vi "ExFileReadNDoMath.vi"() -> ()   [LabVIEW 2010]
panel:
  in  "Full File Name":path
  in  "?":bool
  in  "FileType":u32=67174400
  out "error out":errorcluster
  in  "error in (no error)":errorcluster
  # "ExReadFileNDisplay.vi\nThis example will read in a file of the\nselected data type and display all frames.\nWhen finished viewing data, make sure to\nuse the STOP button to close the display."
  # "File Types:\nSPE = 67371008\nTIF   = 67174400\nPMI  = 67436544"
  # "Browse match pattern is set to *.tif.  Modify this if different file type is needed."
  # "This will properly close\nthe image and\ndeallocate memory."
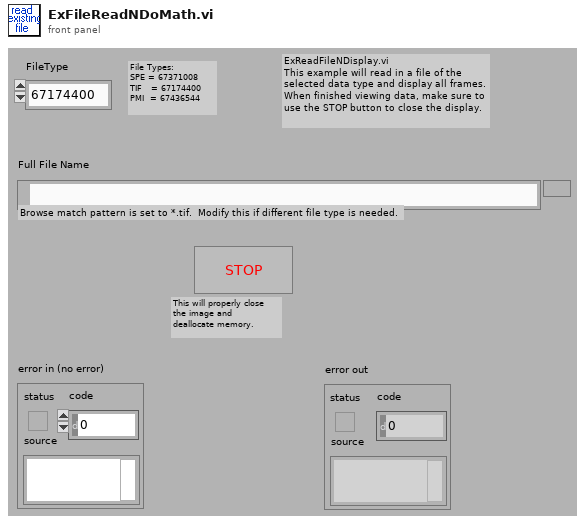
[diagram p1: front panel]
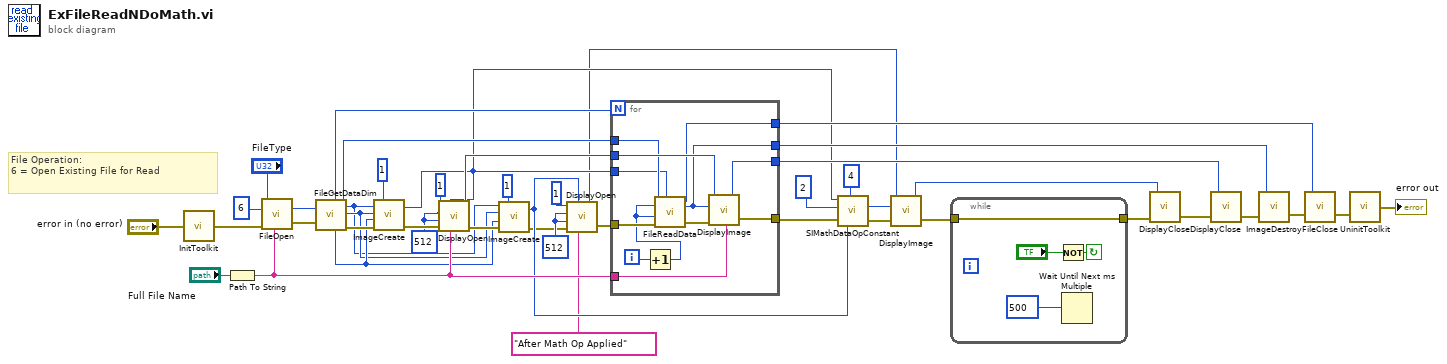
[diagram p0: block diagram]
diagram:
  w13 = 512
  w35 = 512
  # "File Operation:\n6 = Open Existing File for Read"
  n1 = call <userlib>:"InitToolkit.vi"("error in"="error in (no error)") -> ("error out"=w43:errorcluster)
  n2 = Path To String(path="Full File Name") -> (string=w23:string)
  n3 = call <userlib>:"FileOpen.vi"("error in"=w43, "File Operations"=u32 6 ("File Operation"), "FileName"=w23, "File Type"="FileType") -> ("error out"=w41:errorcluster, "File Handle"=w40:u32)
  n4 = call <userlib>:"FileGetDataDim.vi"("File Handle"=w40, "error in"=w41) -> ("Number of Frames"=w37:u32, "Data Type"=w20:u32, "File Handle"=w32:u32, "X dim"=w18:u32, "Y dim"=w19:u32, "error out"=w39:errorcluster)
  n5 = call <userlib>:"ImageCreate.vi"("X dimension"=w18, "Y dimension"=w19, "Data Type"=w20, "error in"=w39, "Number Of Frames"=1) -> ("Image Handle"=w16:u32, "error out"=w38:errorcluster)
  n6 = call <userlib>:"DisplayOpen.vi"("Display Title"=w23, "Image Handle"=w16, "error in"=w38, "Display Height"=w35, "Display Width"=w35, "Display Type"=1) -> ("error out"=w21:errorcluster, "Display Handle"=w33:u32)
  n7 = call <userlib>:"ImageCreate.vi"("X dimension"=w18, "Y dimension"=w19, "Data Type"=w20, "error in"=w21, "Number Of Frames"=1) -> ("Image Handle"=w11:u32, "error out"=w10:errorcluster)
  n8 = call <userlib>:"DisplayOpen.vi"("Display Title"="After Math Op Applied", "Image Handle"=w11, "error in"=w10, "Display Height"=w13, "Display Width"=w13, "Display Type"=1) -> ("error out"=w9:errorcluster, "Display Handle"=w6:u32)
  n9 = for {
    N: w37 -> [_]
    tunnel: w9 -> [w57]
    tunnel: w33 -> [w55]
    tunnel: w32 -> [w54]
    tunnel: w16 -> [w53]
    tunnel: [w50] -> w17
    tunnel: [w49] -> w31
    tunnel: [w48] -> w30
    tunnel: [w47] -> w27
    tunnel: w23 -> [w46]
    i -> [w52]
    n10 = Increment(x=w52) -> (x+1=w51:i32)
    n11 = call <userlib>:"FileReadData.vi"("File Handle"=w54, "Start Frame"=w51, "End Frame"=w51, "error in"=w57, "Image Handle"=w53) -> ("File Handle"=w48:u32, "Image Handle"=w47:u32, "error out"=w56:errorcluster)
    n12 = call <userlib>:"DisplayImage.vi"("error in"=w56, "Title"=w46, "Image Handle"=w47, "Display Handle"=w55) -> ("error out"=w50:errorcluster, "Display Handle"=w49:u32)
  }
  n13 = call <userlib>:"SIMathDataOpConstant.vi"("Data Handle"=w16, "Constant"=2, "Result Handle"=w11, "error in (no error)"=w17, "Operation"=4) -> ("Result Handle"=w7:u32, "error out"=w5:errorcluster)
  n14 = call <userlib>:"DisplayImage.vi"("error in"=w5, "Image Handle"=w7, "Display Handle"=w6) -> ("error out"=w4:errorcluster, "Display Handle"=w1:u32)  [unwired: 1 in]
  n15 = while {
    tunnel: w4 -> [w61]
    tunnel: [w61] -> w3
    stop <- w59 continue-if-true
    n16 = Not(x="?") -> (.not. x?=w59:bool)
    n17 = Wait Until Next ms Multiple(millisecond multiple=500) -> ()  [unwired: 1 out]
  }
  n18 = call <userlib>:"DisplayClose.vi"("error in"=w3, "Display Handle"=w1) -> ("error out"=w2:errorcluster)
  n19 = call <userlib>:"DisplayClose.vi"("error in"=w2, "Display Handle"=w31) -> ("error out"=w29:errorcluster)
  n20 = call <userlib>:"ImageDestroy.vi"("error in"=w29, "Data handle"=w27) -> ("error out"=w28:errorcluster)
  n21 = call <userlib>:"FileClose.vi"("error in"=w28, "File Handle"=w30) -> ("error out"=w26:errorcluster)
  n22 = call <userlib>:"UninitToolkit.vi"("error in"=w26) -> ("error out"=→"error out":errorcluster)
